vi "get_viable_cells.vi"(10 "cell indices":i32[](array[numeric]), 11 "current cell locations (px)":dbl[][](array[numeric])) -> (3 "viable cell locations (px)":dbl[][](array[numeric]))   [LabVIEW 2015]
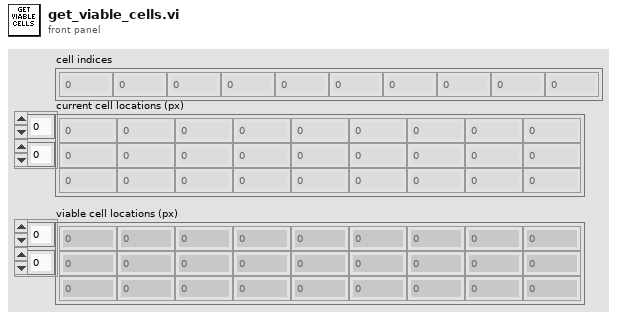
[diagram p1: front panel]
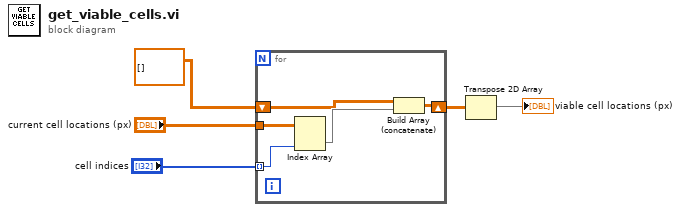
[diagram p0: block diagram]
diagram:
  n1 = for {
    tunnel: "cell indices" -> [w9] mode=indexing
    tunnel: "current cell locations (px)" -> [w10]
    shift-right: [w6] -> w2
    shift-left: dbl[][] [] -> [w7]
    n2 = Index Array(array=w10, index (col)=w9) -> (element=w8:dbl[])  [unwired: 1 in]
    n3 = Build Array (concatenate)(w7, w8) -> (w6:dbl[][])
  }
  n4 = Transpose 2D Array(2D array=w2) -> (transposed array=→"viable cell locations (px)":dbl[][])
